vi "ExcWL2LaserrColor.vi"(1 "Wavelength (380 - 780)":dbl(slide)=380.0 scale=380.0..780.0, 2 "Laser on?":refnum<vi>) -> ()   [LabVIEW 2019]
panel:
  out "Laser on?":bool
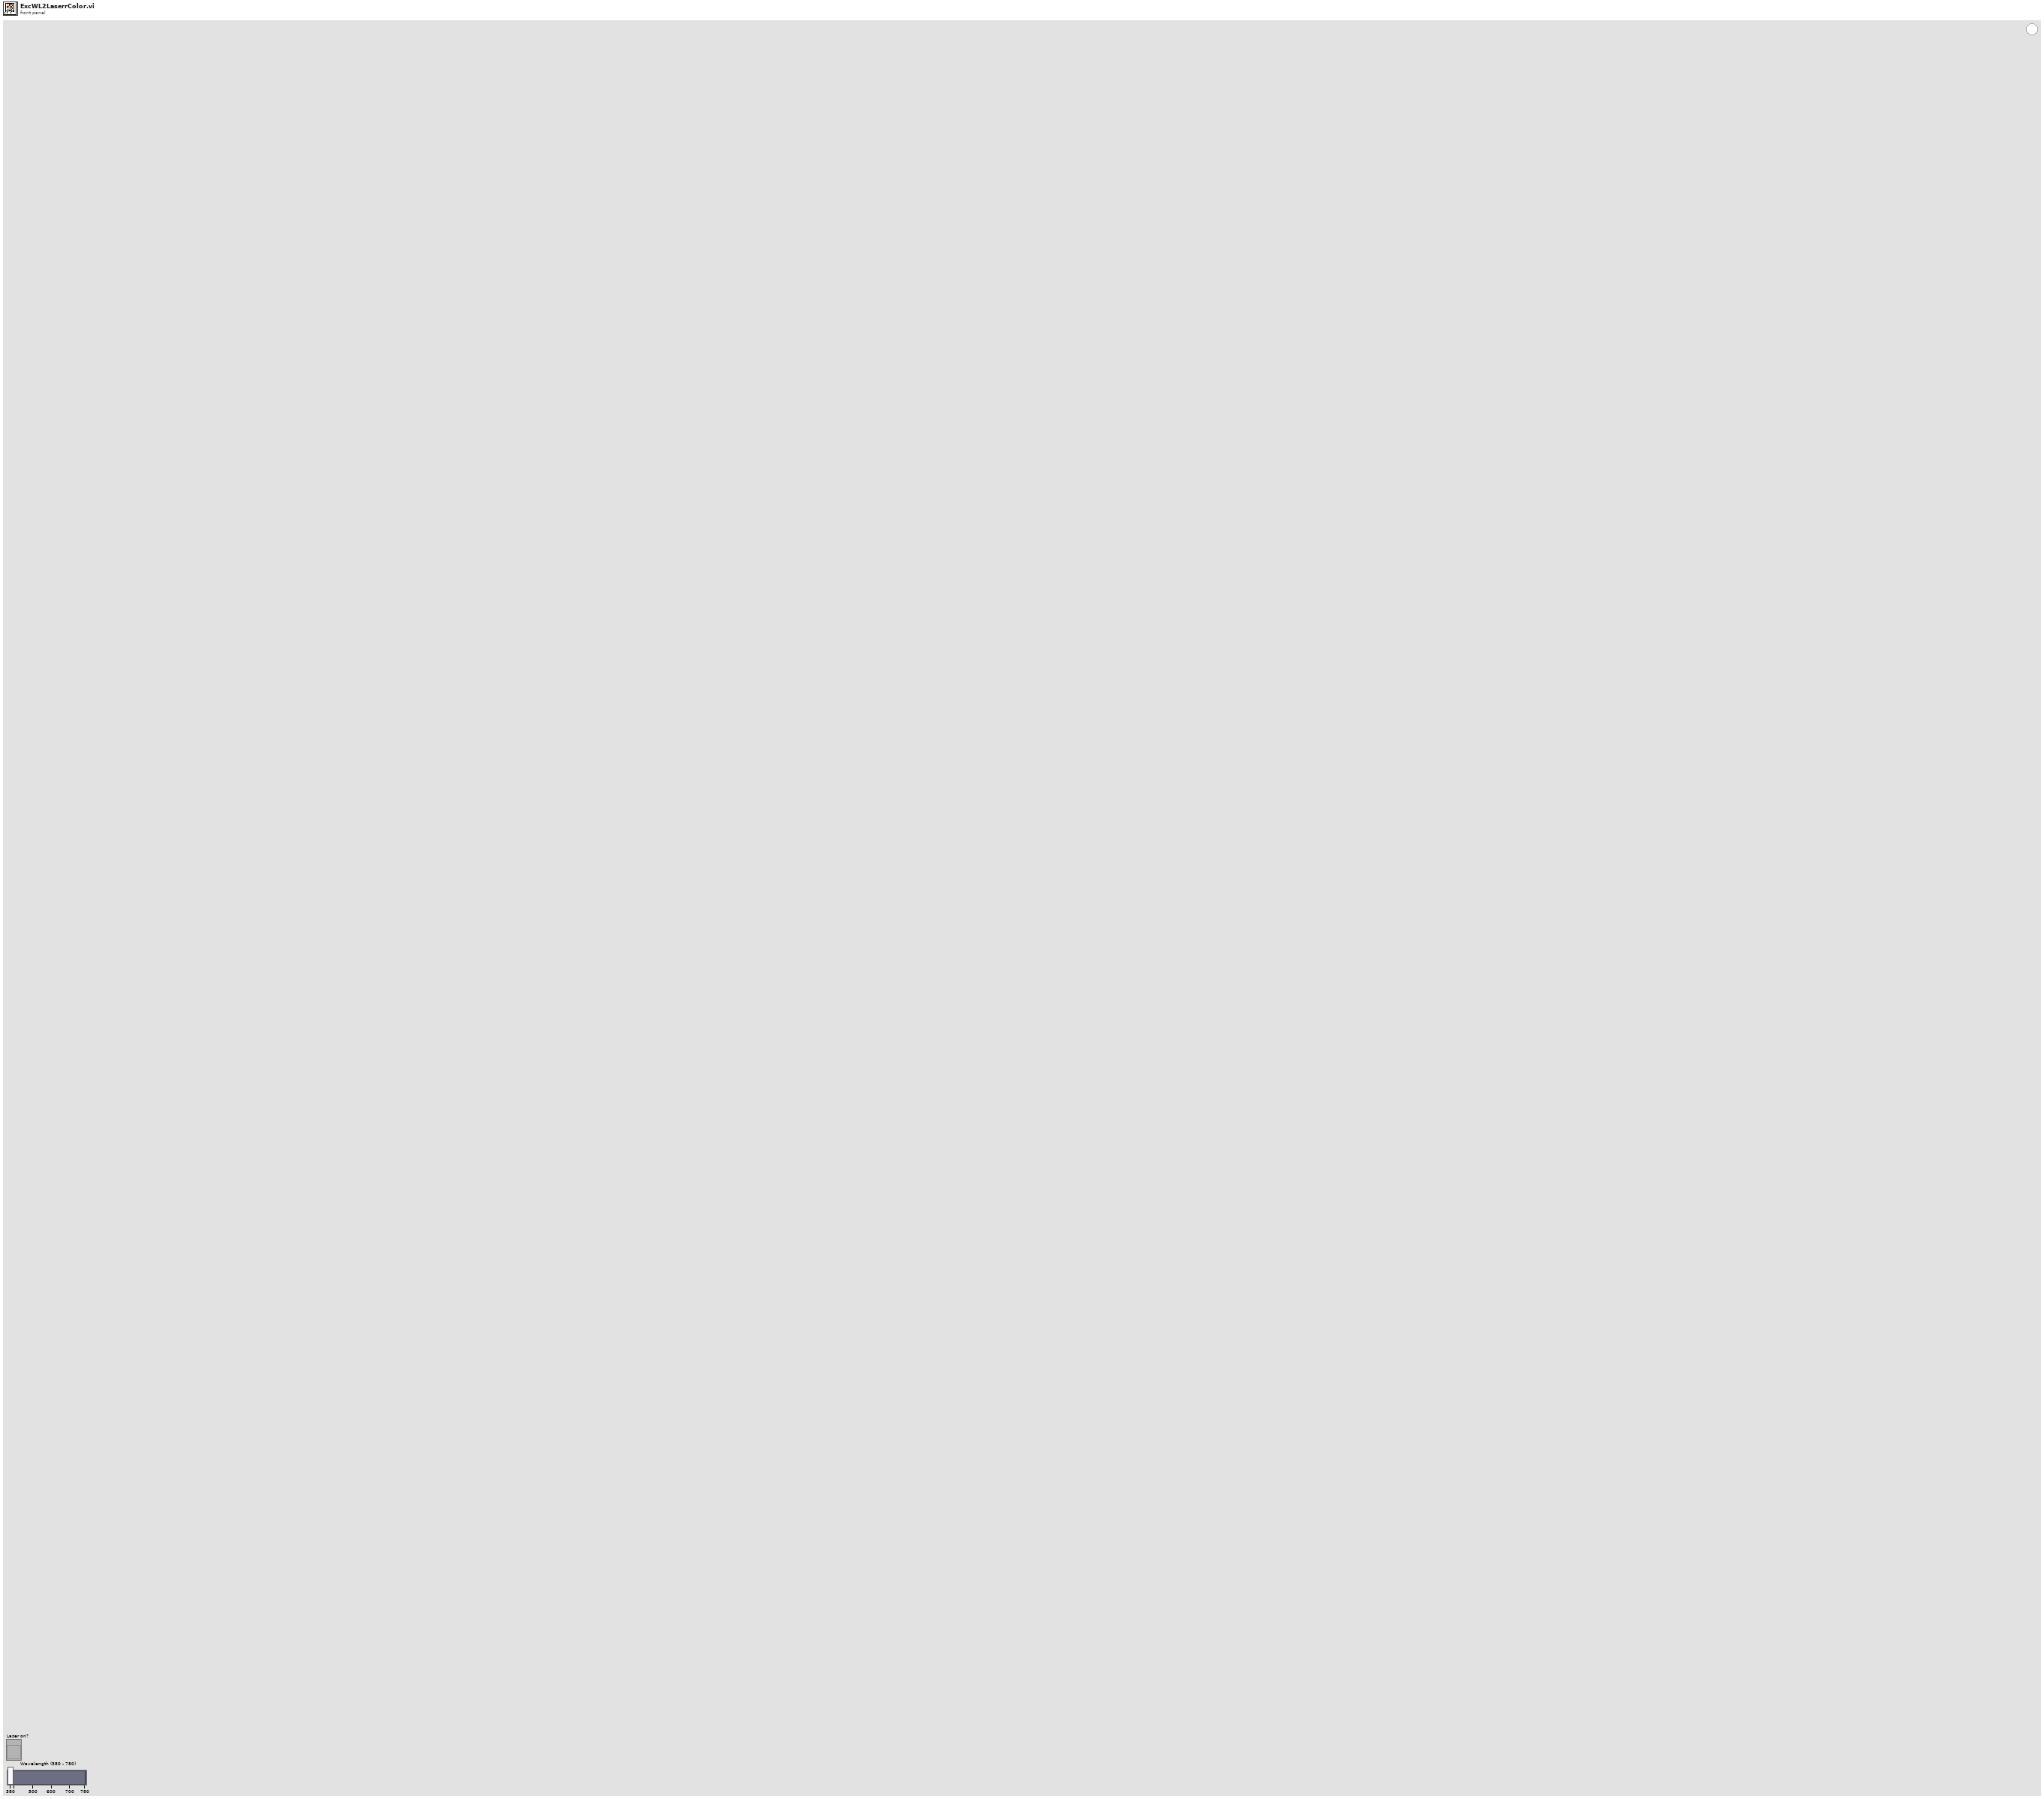
[diagram p1: front panel]
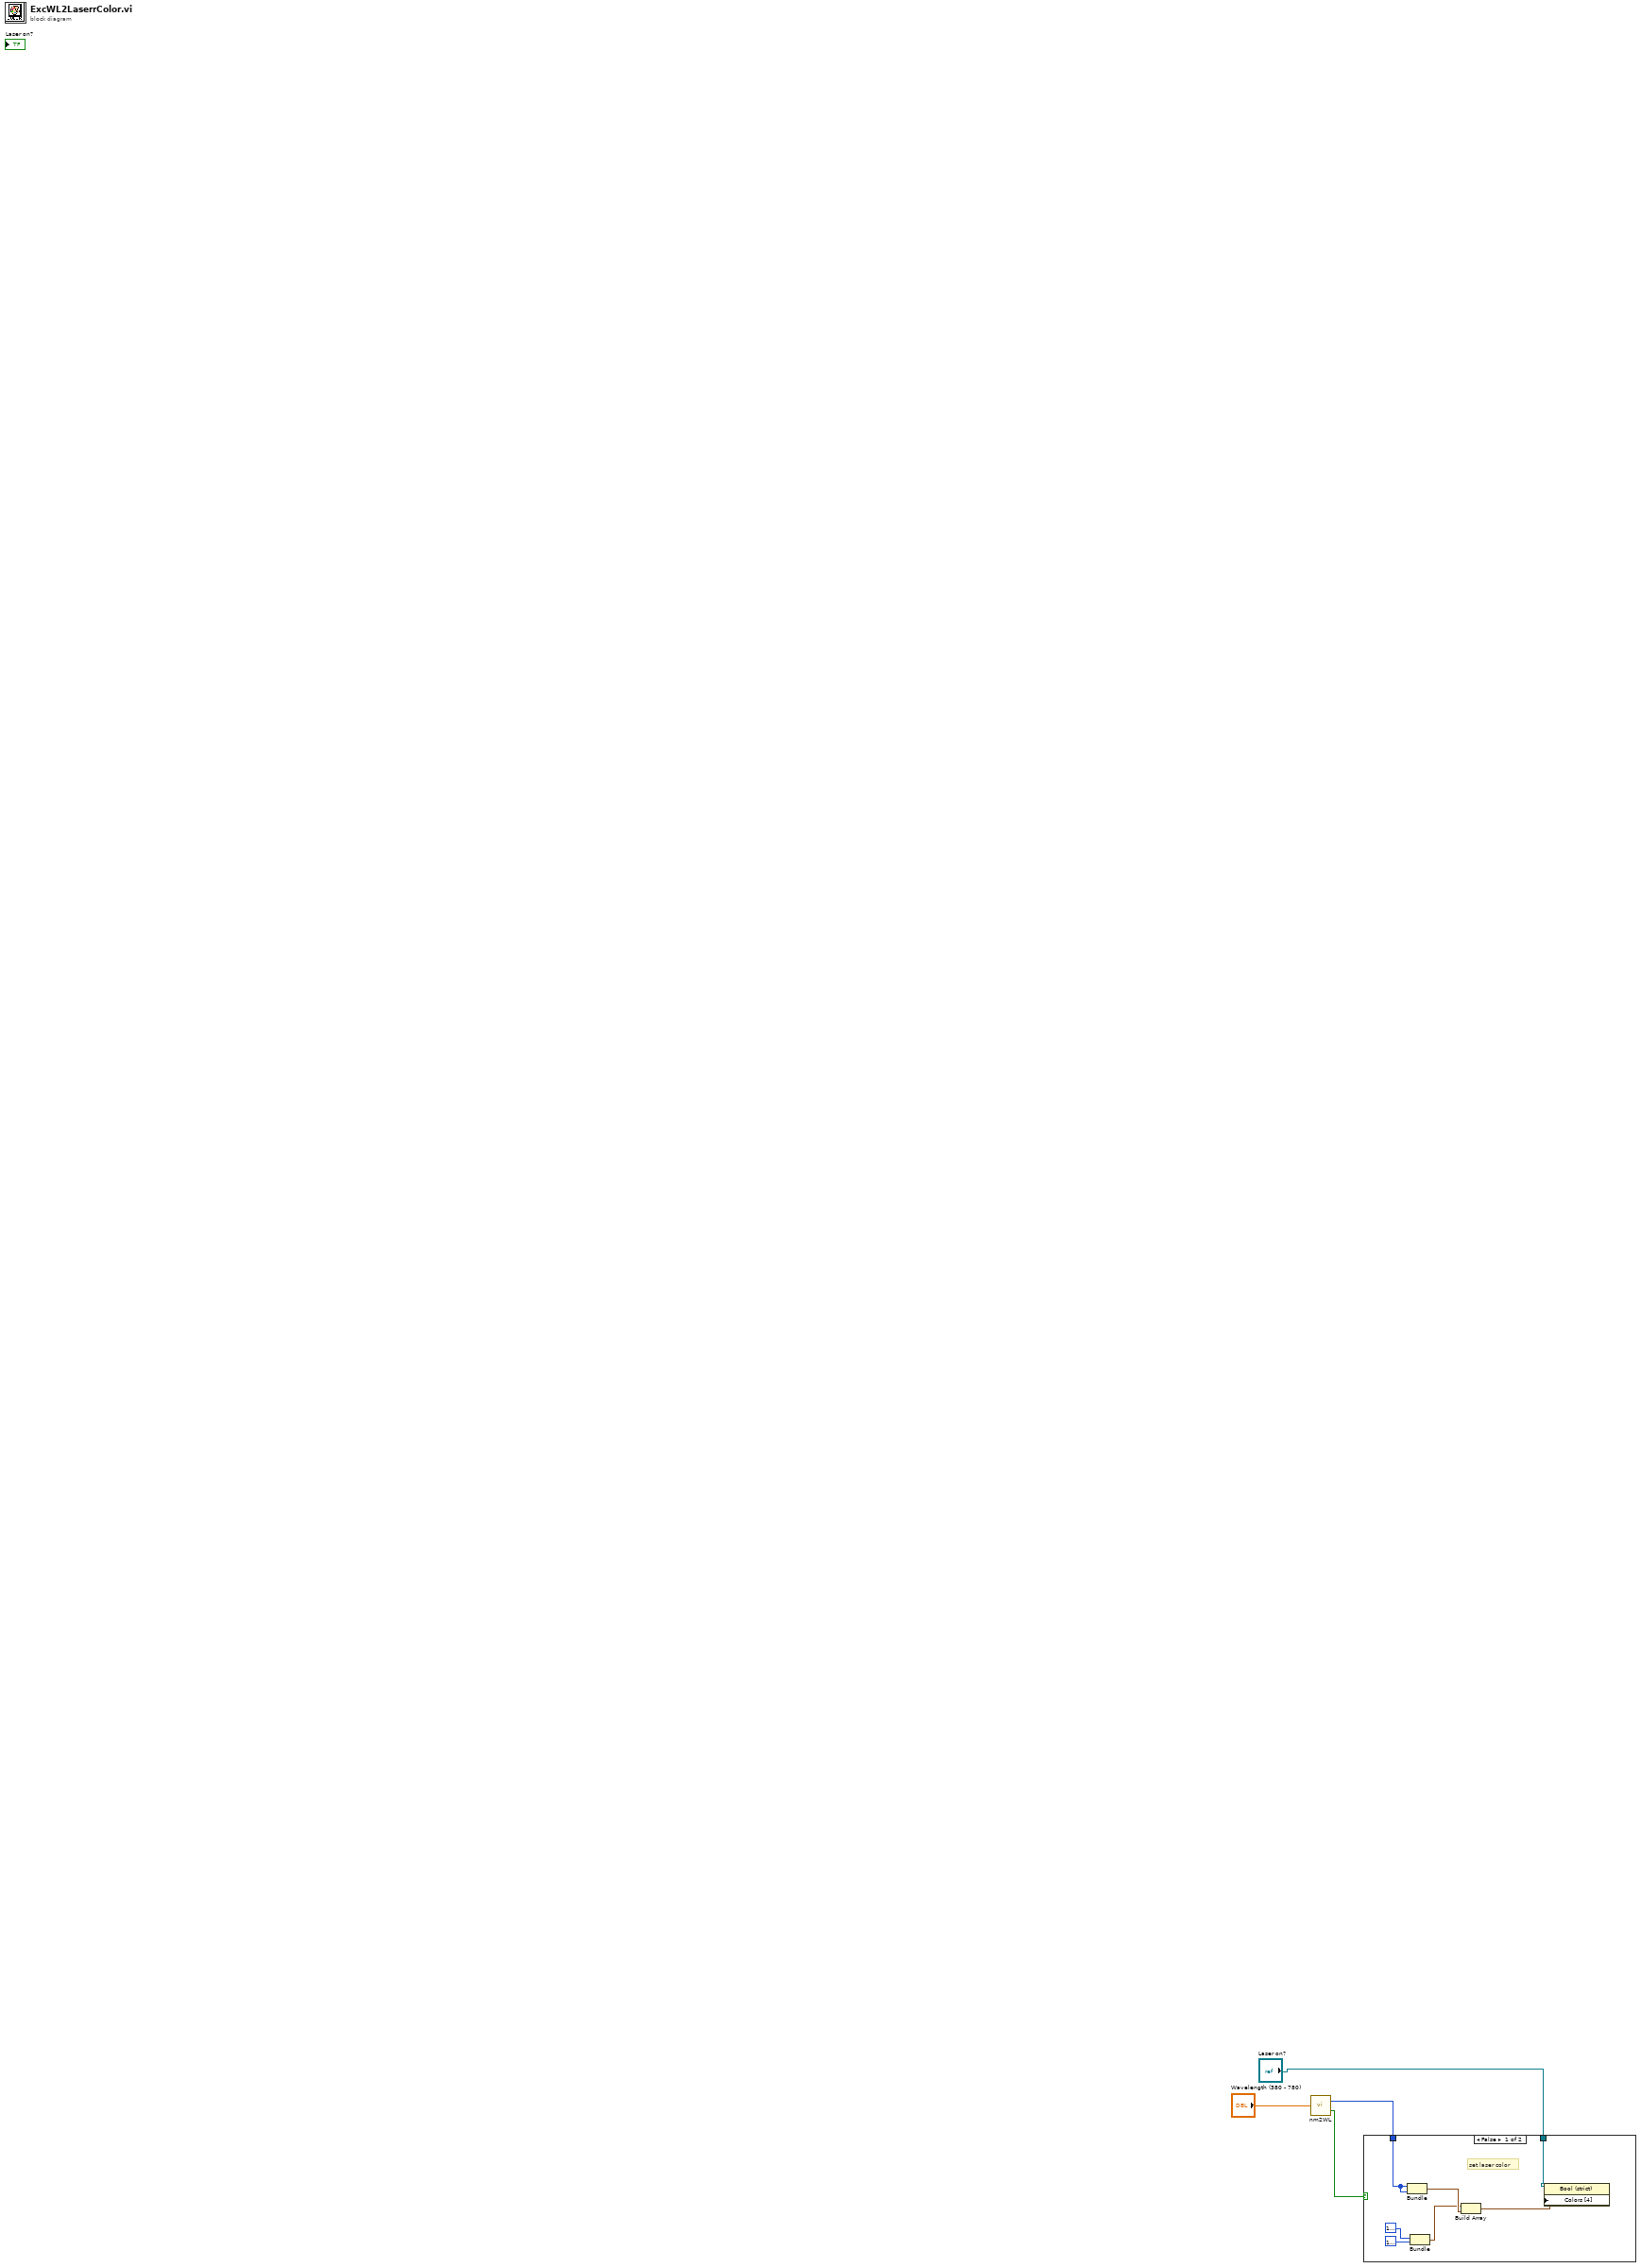
[diagram p0: block diagram]
diagram:
  n1 = call "nm2WL.vi"("Wavelength (380 - 780)"="Wavelength (380 - 780)") -> ("Color"=w4:u32, "Out Of Range"=w3:bool)
  n2 = case shown="False" w3 {
    tunnel: w4 -> [w9 _]
    tunnel: "Laser on?" -> [w5 _]
    frame False {
      # "set laser color"
      n3 = Bundle("Color"=w9, "Color"=w9) -> (w8:cluster{"Color":u32, "Color":u32})  [unwired: 1 in]
      n4 = Bundle(u32 16777216, u32 16777216) -> (w7:cluster{u32, u32})  [unwired: 1 in]
      n5 = Build Array(w7, w8) -> (w6:cluster{"Color":u32, "Color":u32}[])
      n6 = property on="Property Node" class="Bool (strict)"(reference=w5, "Colors [4]"=w6) -> ()  [unwired: 1 in, 2 out]
    }
    frame True {
    }
  }
